vi "Get mode DSP402.vi"(1 "DSP402 in":refnum<class "DSP402.lvclass">) -> (0 "Mode":T1 items=["Undefined"=0, "Profile Position Mode"=1, "Velocity Mode"=2, "Profile Velocity Mode"=3, "Torque Profile Mode"=4, "Homing Mode"=6, "Interpolated Position Mode"=7])   [LabVIEW 2017, in "canopen.lvlib" / "DSP402.lvclass"]
uses:
  DSP402.lvclass
  DriveMode.ctl
  DSP402.lvclass/DSP402.ctl
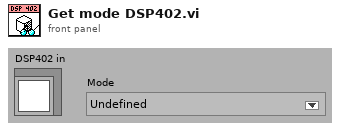
[diagram p1: front panel]
types:
  T1 = typedef "canopen.lvlib/DSP402.lvclass/DriveMode.ctl" = i8
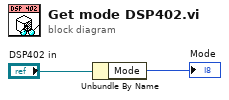
[diagram p0: block diagram]
diagram:
  n1 = Unbundle By Name("DSP402 in") -> ("Mode"=→"Mode":T1)
